vi "IPC-Core-DAQModule.vi"(0 "DataQRef":refnum<queue>, 5 "DaqQRef":refnum<queue>, 7 "6133QRef":refnum<queue>, 9 "ErrorQRef":refnum<queue>, 11 "error in":errorcluster) -> (15 "错误输出":errorcluster)   [LabVIEW 2014]
uses:
  Configuration-Global.vi
panel:
  out "x-y":u32
  out "毫秒计时值":u32
  out "最小公倍数 2":i32
  in  "采样率":i32[](array[numeric])=[32000, 32000, 32000, 32000, 32000, 32000, 80000, 80000]
  out "DAQ Deamo is Running":bool
  in  "开关":bool=TRUE
  out "Daq::Initialize":dbl[](array[numeric])
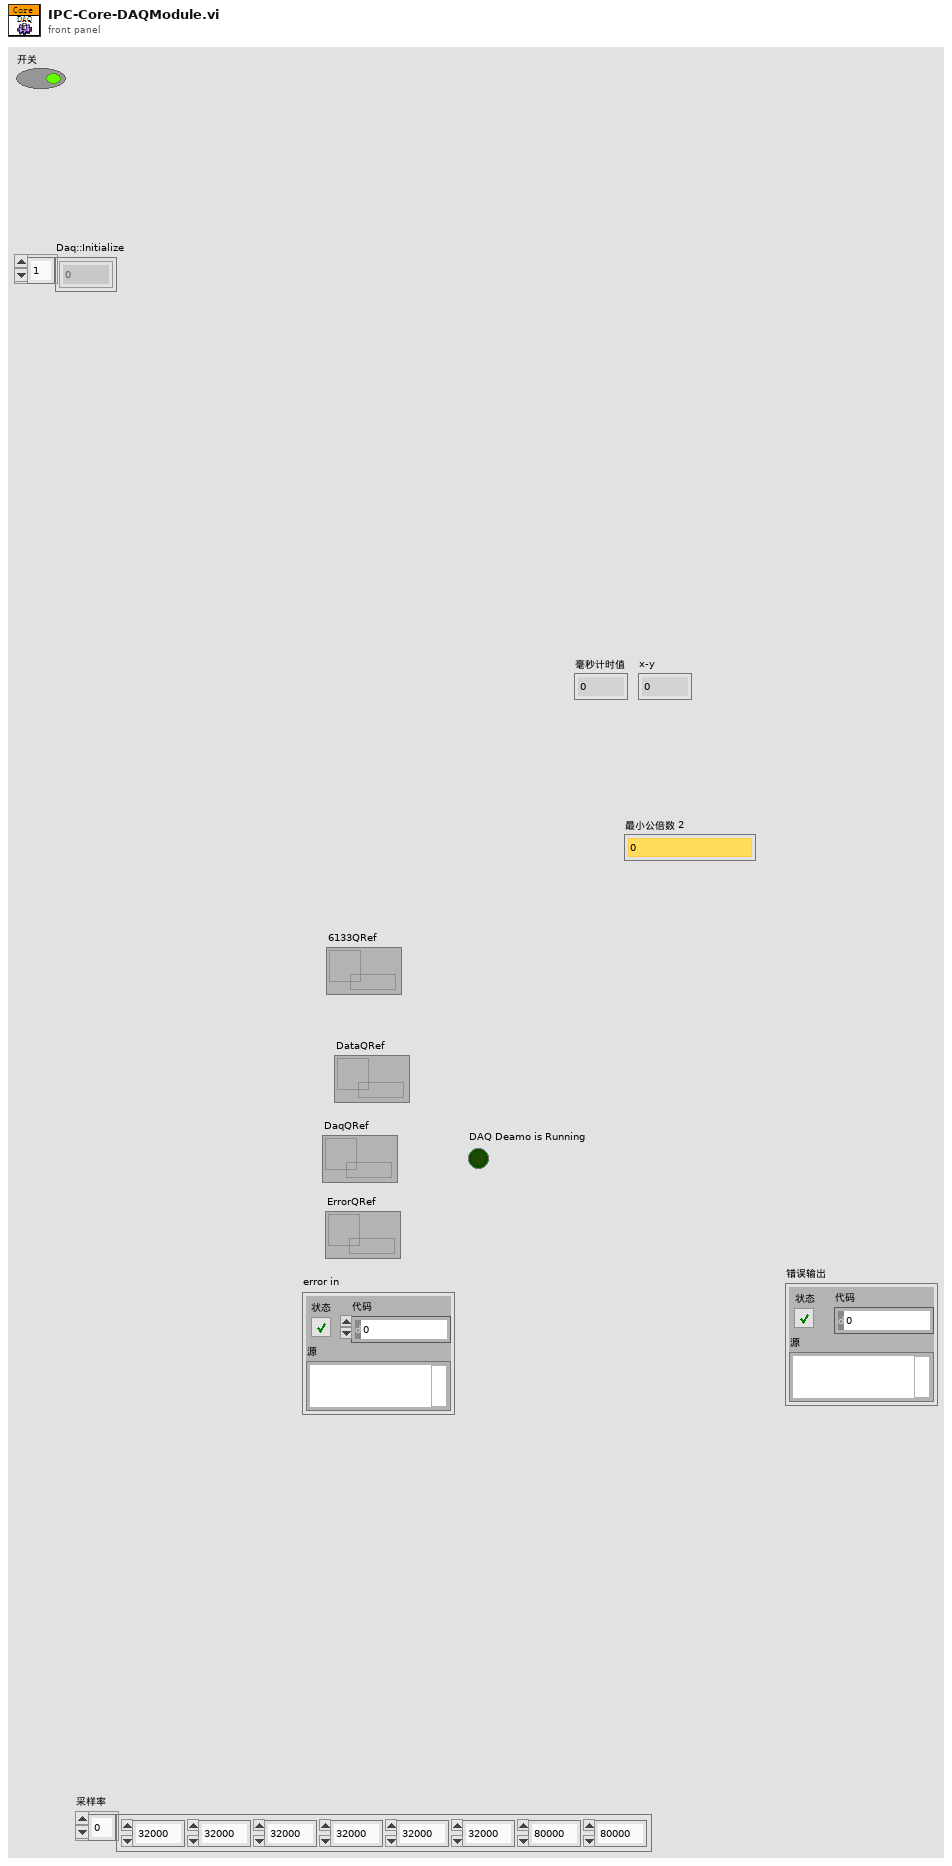
[diagram p1: front panel]
types:
  T1 = cluster{string, "seconds since 1Jan1904":timestamp, "data":dbl[][]}
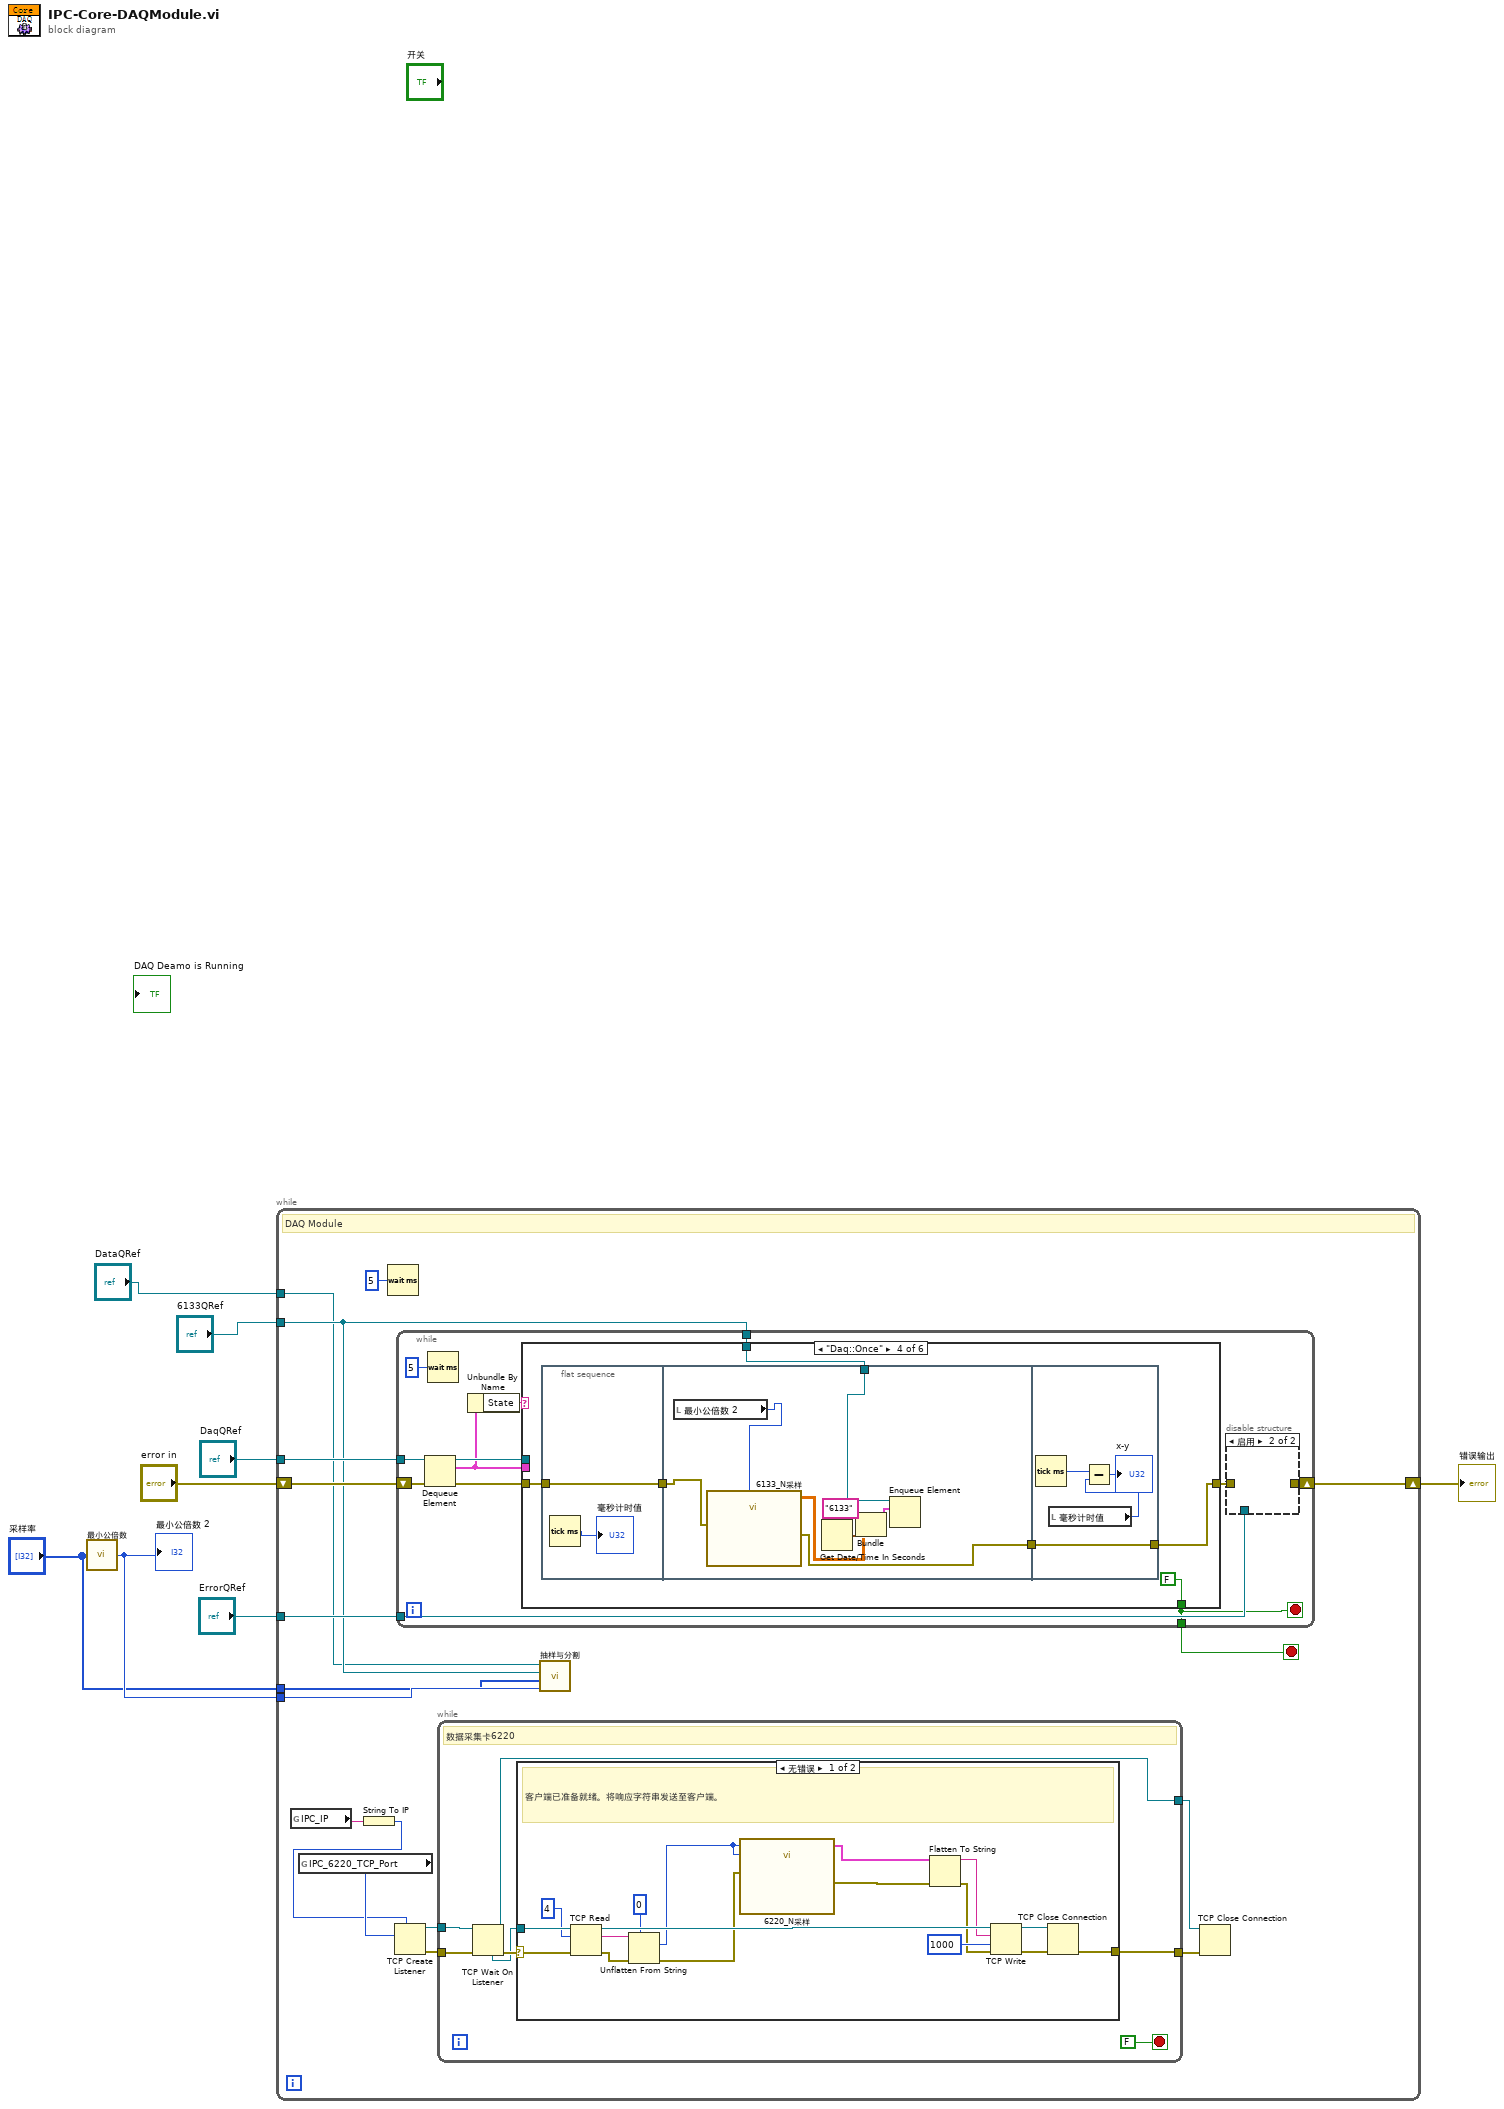
[diagram p0: block diagram]
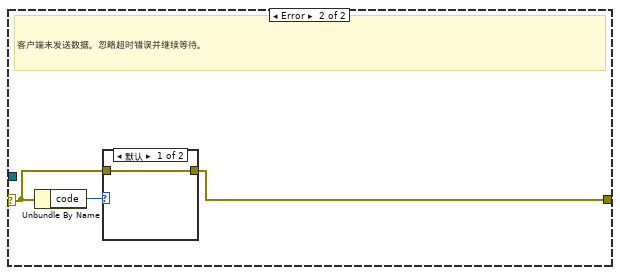
[diagram p2: hidden frame]
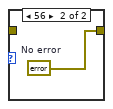
[diagram p3: hidden frame]
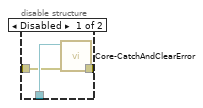
[diagram p4: hidden frame]
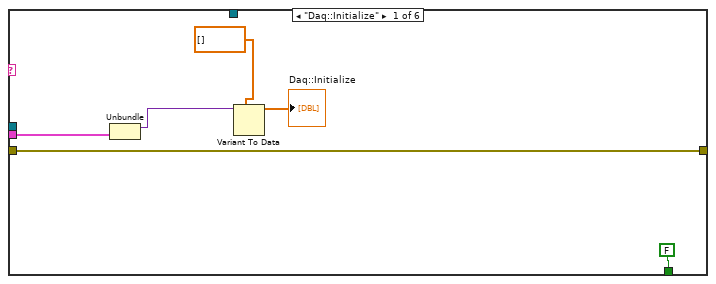
[diagram p5: hidden frame]
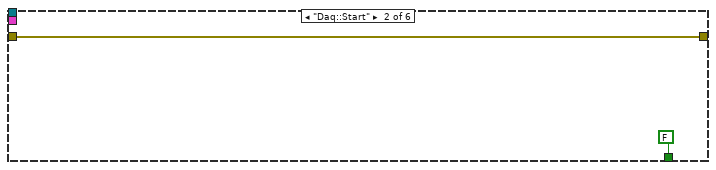
[diagram p6: hidden frame]
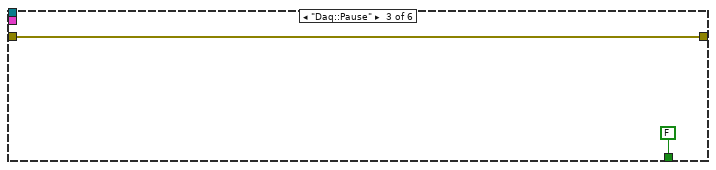
[diagram p7: hidden frame]
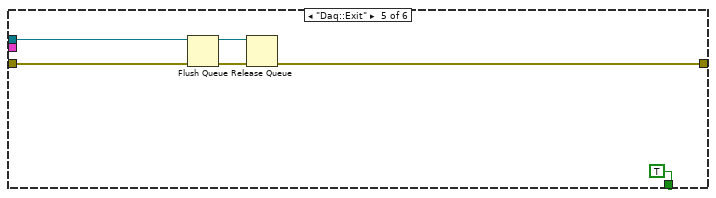
[diagram p8: hidden frame]
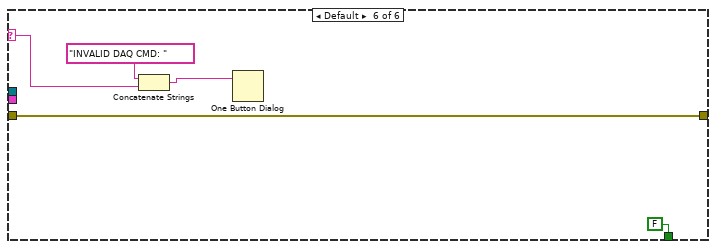
[diagram p9: hidden frame]
diagram:
  n1 = call "最小公倍数.vi"("采样率"="采样率") -> ("最小公倍数 2"=w3:i32)
  "最小公倍数 2" <- w3
  n2 = while {
    shift-right: [w9] -> w5
    shift-left: "error in" -> [w22]
    tunnel: "ErrorQRef" -> [w21]
    tunnel: "DaqQRef" -> [w24]
    tunnel: "DataQRef" -> [w13]
    tunnel: "6133QRef" -> [w18]
    tunnel: w3 -> [w20]
    tunnel: "采样率" -> [w19]
    stop <- w23 stop-if-true
    # "DAQ Module"
    n3 = global read "Configuration-Global.vi" "IPC_IP"() -> (w11:string)
    n4 = global read "Configuration-Global.vi" "IPC_6220_TCP_Port"() -> (w12:i32)
    n5 = String To IP(1:w11) -> (0:w10:u32)
    n6 = Wait (ms)(milliseconds to wait=u32 5 ("等待时间（毫秒）")) -> ()  [unwired: 1 out]
    n7 = TCP Create Listener(7:w10, 10:w12) -> (0:w14:errorcluster, 3:w15:refnum<k5>)  [unwired: 3 in, 1 out]
    n8 = while {
      tunnel: w21 -> [w61]
      tunnel: w24 -> [w58]
      tunnel: [w57] -> w23
      shift-right: [w62] -> w9
      shift-left: w22 -> [w66]
      tunnel: w18 -> [w55]
      stop <- w57 stop-if-true
      n9 = Dequeue Element(queue=w58, error in (no error)=w66) -> (queue out=w63:refnum<queue>, element=w59:cluster{"Data":variant, "State":string}, error out=w65:errorcluster)  [unwired: 1 in, 1 out]
      n10 = Wait (ms)(milliseconds to wait=u32 5 ("等待时间（毫秒）")) -> ()  [unwired: 1 out]
      n11 = Unbundle By Name(w59) -> ("State"=w64:string)
      n12 = case shown="\"Daq::Once\"" w64 {
        selector: w64 -> [_ _ _ _ _ w107]
        tunnel: w65 -> [w75 w76 w78 w85 w103 w110]
        tunnel: [w75 w76 w78 w84 w102 w110] -> w60
        tunnel: w63 -> [_ _ _ _ w101 _]
        tunnel: w59 -> [w74 _ _ _ _ _]
        tunnel: [FALSE FALSE FALSE FALSE TRUE FALSE] -> w57
        tunnel: w55 -> [_ _ _ w82 _ _]
        frame "Daq::Initialize" {
          n13 = Unbundle(w74) -> ("Data"=w73:variant)  [unwired: 1 out]
          n14 = Variant To Data(type=dbl[] [], Variant=w73) -> (data=→"Daq::Initialize":dbl[])  [unwired: 1 in, 1 out]
        }
        frame "Daq::Start" {
        }
        frame "Daq::Pause" {
        }
        frame "Daq::Once" {
          n15 = flat-sequence {
            tunnel: w85 -> [w87]
            tunnel: [w87] -> w80
            tunnel: w82 -> [w94]
            tunnel: [w88] -> w81
            tunnel: w80 -> [w89]
            tunnel: [w99] -> w84
            tunnel: w81 -> [w99]
            frame #0 {
              n16 = Tick Count (ms)() -> (millisecond timer value=→"毫秒计时值":u32)
            }
            frame #1 {
              n17 = local read "最小公倍数 2"() -> (w95:i32)
              n18 = call "6133_N采样.vi"("率"=w95, "采样数"=w95, "error in"=w89) -> ("data"=w91:dbl[][], "error out"=w88:errorcluster)  [unwired: 15 in]
              n19 = Get Date/Time In Seconds() -> (seconds since 1Jan1904=w92:timestamp)
              n20 = Bundle("6133", "seconds since 1Jan1904"=w92, "data"=w91) -> (w90:T1)  [unwired: 1 in]
              n21 = Enqueue Element(queue=w94, element=w90) -> ()  [unwired: 2 in, 3 out]
            }
            frame #2 {
              n22 = Tick Count (ms)() -> (millisecond timer value=w98:u32)
              n23 = local read "毫秒计时值"() -> (w97:u32)
              n24 = Subtract(x=w98, y=w97) -> (x-y=→"x-y":u32)
            }
          }
        }
        frame "Daq::Exit" {
          n25 = Flush Queue(queue=w101, error in (no error)=w103) -> (queue out=w105:refnum<queue>, error out=w104:errorcluster)  [unwired: 1 out]
          n26 = Release Queue(queue=w105, error in (no error)=w104) -> (error out=w102:errorcluster)  [unwired: 1 in, 2 out]
        }
        frame Default {
          n27 = Concatenate Strings("INVALID DAQ CMD: ", w107) -> (w108:string)
          n28 = One Button Dialog(message=w108) -> ()  [unwired: 1 in, 1 out]
        }
      }
      n29 = disable-structure shown="启用" {
        disable-tunnel: [w69 _] -> w62
        disable-tunnel: w61 -> [w68 _]
        disable-tunnel: w60 -> [w67 _]
        frame Disabled {
          n30 = call "Core-CatchAndClearError.vi"("error in (no error)"=w67, "ErrorQ"=w68) -> ("error out"=w69:errorcluster)  [unwired: 7 in]
        }
        frame Enabled {
        }
      }
    }
    n31 = while {
      tunnel: w15 -> [w32]
      tunnel: [w27] -> w17
      tunnel: w14 -> [w31]
      tunnel: [w28] -> w16
      stop <- FALSE stop-if-true
      # "数据采集卡6220"
      n32 = TCP Wait On Listener(8:w31, 11:w32) -> (0:w30:errorcluster, 3:w27:refnum<k5>, 4:w26:refnum<k5>)  [unwired: 2 in, 2 out]
      n33 = case shown="无错误" w30 {
        selector: w30 -> [w46 w51]
        tunnel: [w49 w50] -> w28
        tunnel: w26 -> [w45 _]
        frame No Error {
          # "客户端已准备就绪。将响应字符串发送至客户端。"
          n34 = TCP Read(connection ID=w45, bytes to read=4 ("读取的字节"), error in (no error)=w46) -> (connection ID out=w44:refnum<k5>, data out=w34:string, error out=w42:errorcluster)  [unwired: 2 in]
          n35 = Unflatten From String(type=0 ("读取的字节"), binary string=w34, error in (no error)=w42) -> (value=w40:i32, error out=w38:errorcluster)  [unwired: 2 in, 1 out]
          n36 = call "6220_N采样.vi"("率"=w40, "采样数"=w40, "error in"=w38) -> ("6220"=w33:cluster{"时间":timestamp, "数据":sgl[][]}, "error out"=w37:errorcluster)  [unwired: 15 in]
          n37 = Flatten To String(anything=w33, error in (no error)=w37) -> (data string=w36:string, error out=w35:errorcluster)  [unwired: 2 in, 1 out]
          n38 = TCP Write(connection ID=w44, data in=w36, error in (no error)=w35, 9:1000 ("超时毫秒(25000)")) -> (connection ID out=w48:refnum<k5>, error out=w39:errorcluster)  [unwired: 1 out]
          n39 = TCP Close Connection(connection ID=w48, error in (no error)=w39) -> (error out=w49:errorcluster)  [unwired: 1 in, 1 out]
        }
        frame Error {
          # "客户端未发送数据。忽略超时错误并继续等待。"
          n40 = Unbundle By Name(w51) -> ("code"=w52:i32)
          n41 = case shown="默认" w52 {
            tunnel: w51 -> [w53 _]
            tunnel: [w53 w54] -> w50
            frame Default {
            }
            frame 56 {
              w54 = errorcluster {"status"=FALSE, "code"=0, "source"=""}  # No error
            }
          }
        }
      }
    }
    n42 = call "抽样与分割.vi"("采样数"=w20, "采样率"=w19, "6133队列"=w18, "DataQRef"=w13) -> ()  [unwired: 8 in]
    n43 = TCP Close Connection(connection ID=w17, error in (no error)=w16) -> ()  [unwired: 1 in, 2 out]
  }
  "错误输出" <- w5
